vi "rename sequence.vi"(8 "error in (no error)":errorcluster, 9 "new sequence name":string, 10 "old sequence name":string, 11 "Simple Sequencer TBM configuration in":refnum<class "Simple Sequencer TBM configuration.lvclass">) -> (0 "error out":errorcluster, 3 "Simple Sequencer TBM configuration out":refnum<class "Simple Sequencer TBM configuration.lvclass">)   [LabVIEW 2015, in "Simple Sequencer TBM configuration.lvclass"]
uses:
  Simple Sequencer TBM configuration.lvclass
  Simple Sequencer TBM configuration.lvclass/Simple Sequencer TBM configuration.ctl
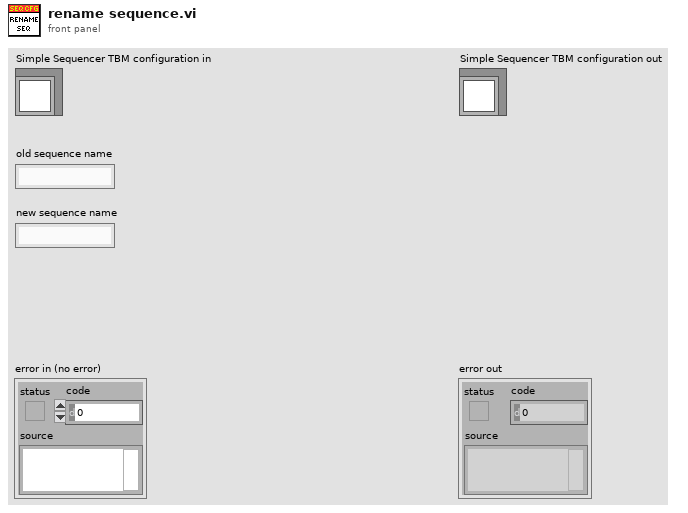
[diagram p1: front panel]
types:
  T1 = typedef "Simple Sequencer TBM configuration.lvclass/sequence definition.ctl" = cluster{"sequence name":string, "action configs":refnum<class "action configuration.lvclass">[]}
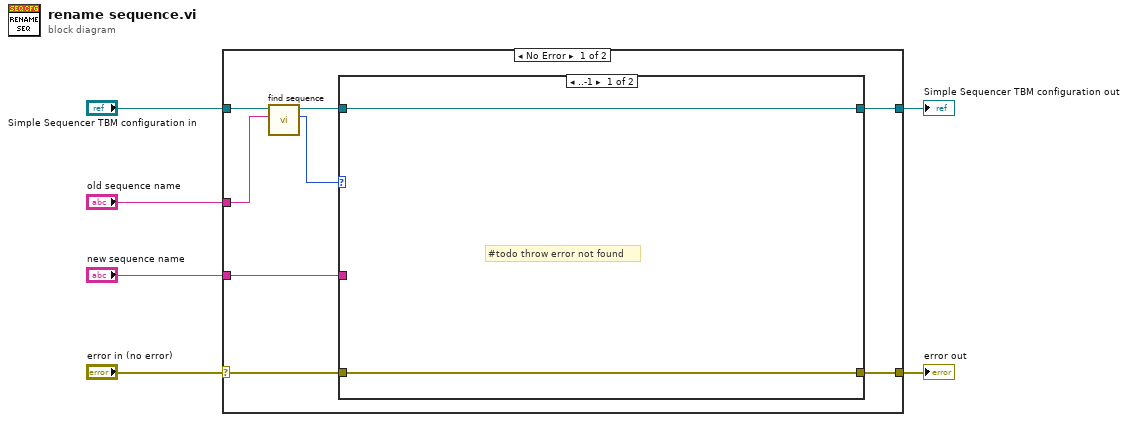
[diagram p0: block diagram]
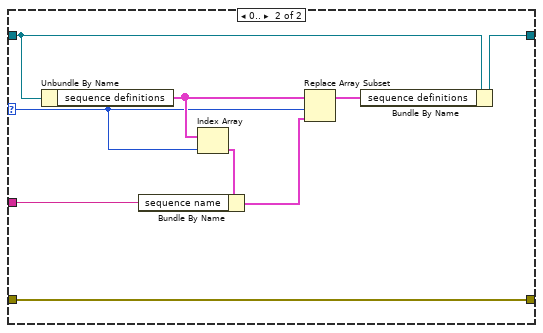
[diagram p2: hidden frame]
diagram:
  n1 = case shown="No Error" "error in (no error)" {
    selector: "error in (no error)" -> [w10 w27]
    tunnel: [w9 w27] -> w5
    tunnel: [w7 w26] -> w3
    tunnel: "Simple Sequencer TBM configuration in" -> [w14 w26]
    tunnel: "old sequence name" -> [w13 _]
    tunnel: "new sequence name" -> [w8 _]
    frame No Error {
      n2 = call "find sequence.vi"("sequence name"=w13, "Simple Sequencer TBM configuration in"=w14) -> ("index"=w11:i32, "Simple Sequencer TBM configuration out"=w12:refnum<class "Simple Sequencer TBM configuration.lvclass">)  [unwired: 8 in]
      n3 = case shown="..-1" w11 {
        selector: w11 -> [_ w21]
        tunnel: w12 -> [w15 w19]
        tunnel: w10 -> [w16 w25]
        tunnel: [w16 w25] -> w9
        tunnel: w8 -> [_ w23]
        tunnel: [w15 w17] -> w7
        frame ..-1 {
          # "#todo throw error not found"
        }
        frame 0.. {
          n4 = Unbundle By Name(w19) -> ("sequence definitions"=w22:T1[])
          n5 = Index Array(array=w22, index=w21) -> (element=w24:T1)
          n6 = Bundle By Name(cluster=w24, "sequence name"=w23) -> (w20:T1)
          n7 = Replace Array Subset(array=w22, new element=w20, index=w21) -> (w18:T1[])
          n8 = Bundle By Name(cluster=w19, "sequence definitions"=w18) -> (w17:refnum<class "Simple Sequencer TBM configuration.lvclass">)
        }
      }
    }
    frame Error {
    }
  }
  "error out" <- w5
  "Simple Sequencer TBM configuration out" <- w3
